vi "Dual_image_snap.vi"() -> ()   [LabVIEW 2013]
uses:
  <vilib>/DAQmx/create/channels.llb/DAQmx Create Channel (CO-Pulse Generation-Frequency).vi
  <vilib>/DAQmx/configure/timing.llb/DAQmx Timing (Implicit).vi
  <vilib>/vision/driver/NI_Vision_Acquisition_Software.lvlib
  <resource>/objmgr/imaqdx.rc
  <resource>/objmgr/daqmx.rc
panel:
  out "Snap Counter":u32
  in  "Snap":bool
  in  "Gain 2":dbl(slide)=575.0 min=350.0 max=1000.0 step=1.0 scale=350.0..1000.0
  in  "VR2":dbl(slide)=65.0 min=0.0 max=255.0 step=1.0 scale=0.0..255.0
  in  "VR1":dbl(slide)=60.0 min=0.0 max=255.0 step=1.0 scale=0.0..255.0
  in  "UB2":dbl(slide)=160.0 min=0.0 max=255.0 step=1.0 scale=0.0..255.0
  in  "UB1":dbl(slide)=165.0 min=0.0 max=255.0 step=1.0 scale=0.0..255.0
  in  "Shutter":dbl(slide)=4095.0 min=0.0 max=4095.0 step=1.0 scale=4.095..4095.0 scale format="%#.0f"
  in  "Brightness":dbl(slide)=100.0 min=0.0 max=255.0 step=1.0 scale=0.0..255.0
  in  "Gain":dbl(slide)=600.0 min=350.0 max=1000.0 step=1.0 scale=350.0..1000.0
  in  "Test Description":string="test"
  in  "Storage Directory":path=path "C:/Users/Regen/Desktop/Users/Ryan Gergely/3D_DIC"
  out "Image 2":T1(plugin-control)
  out "Buffer Number 2":u32
  out "Frame Rate 2":dbl
  in  "Camera Name 2":refnum<k21>="cam2" caption="IMAQdx Session"
  in  "Pule Frequency":dbl=2.0 format="%.1f"
  out "Actual Duty Cycle":dbl
  out "Actual Pulse Frequency":dbl
  in  "Stop":bool
  in  "Start Trigger Mode":bool
  out "Frame Rate 1":dbl
  out "Buffer Number 1":u32
  in  "Camera Name 1":refnum<k21>="cam1" caption="IMAQdx Session"
  out "Image 1":T1(plugin-control)
  # "1) Set Test Description and Storage Directory"
  # "2) Select Cameras"
  # "3) Start VI"
  # "4) Set Frequency and Exposure and White Balance\n(Before Start Trigger)"
  # "5)"
  # "6) Stop When Done"
  # "Exposure Settings - Both Cameras"
  # "White Balance - Camera1"
  # "White Balance - Camera2"
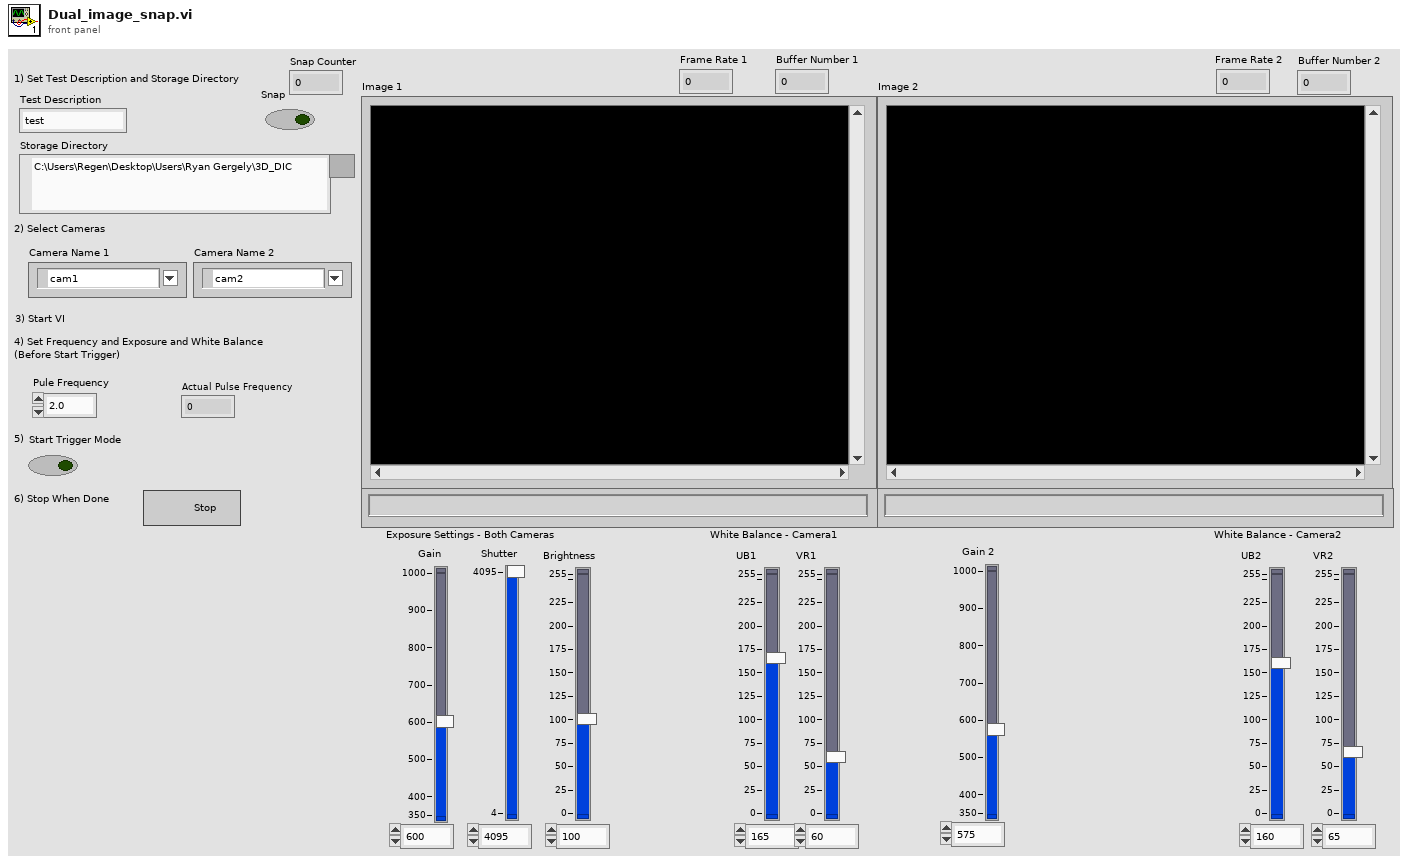
[diagram p1: front panel]
types:
  T1 = typedef "IMAQ Image.ctl" = refnum<image>
  T2 = typedef "IMAQdx.ctl" = refnum<k21>
  T3 = enum16{"open", "replace", "create", "open or create", "replace or create", "replace or create with confirmation"}
  T4 = cluster{"Trigger Mode":u32, "Trigger Activation":u32, "Timeout (ms)":u32}
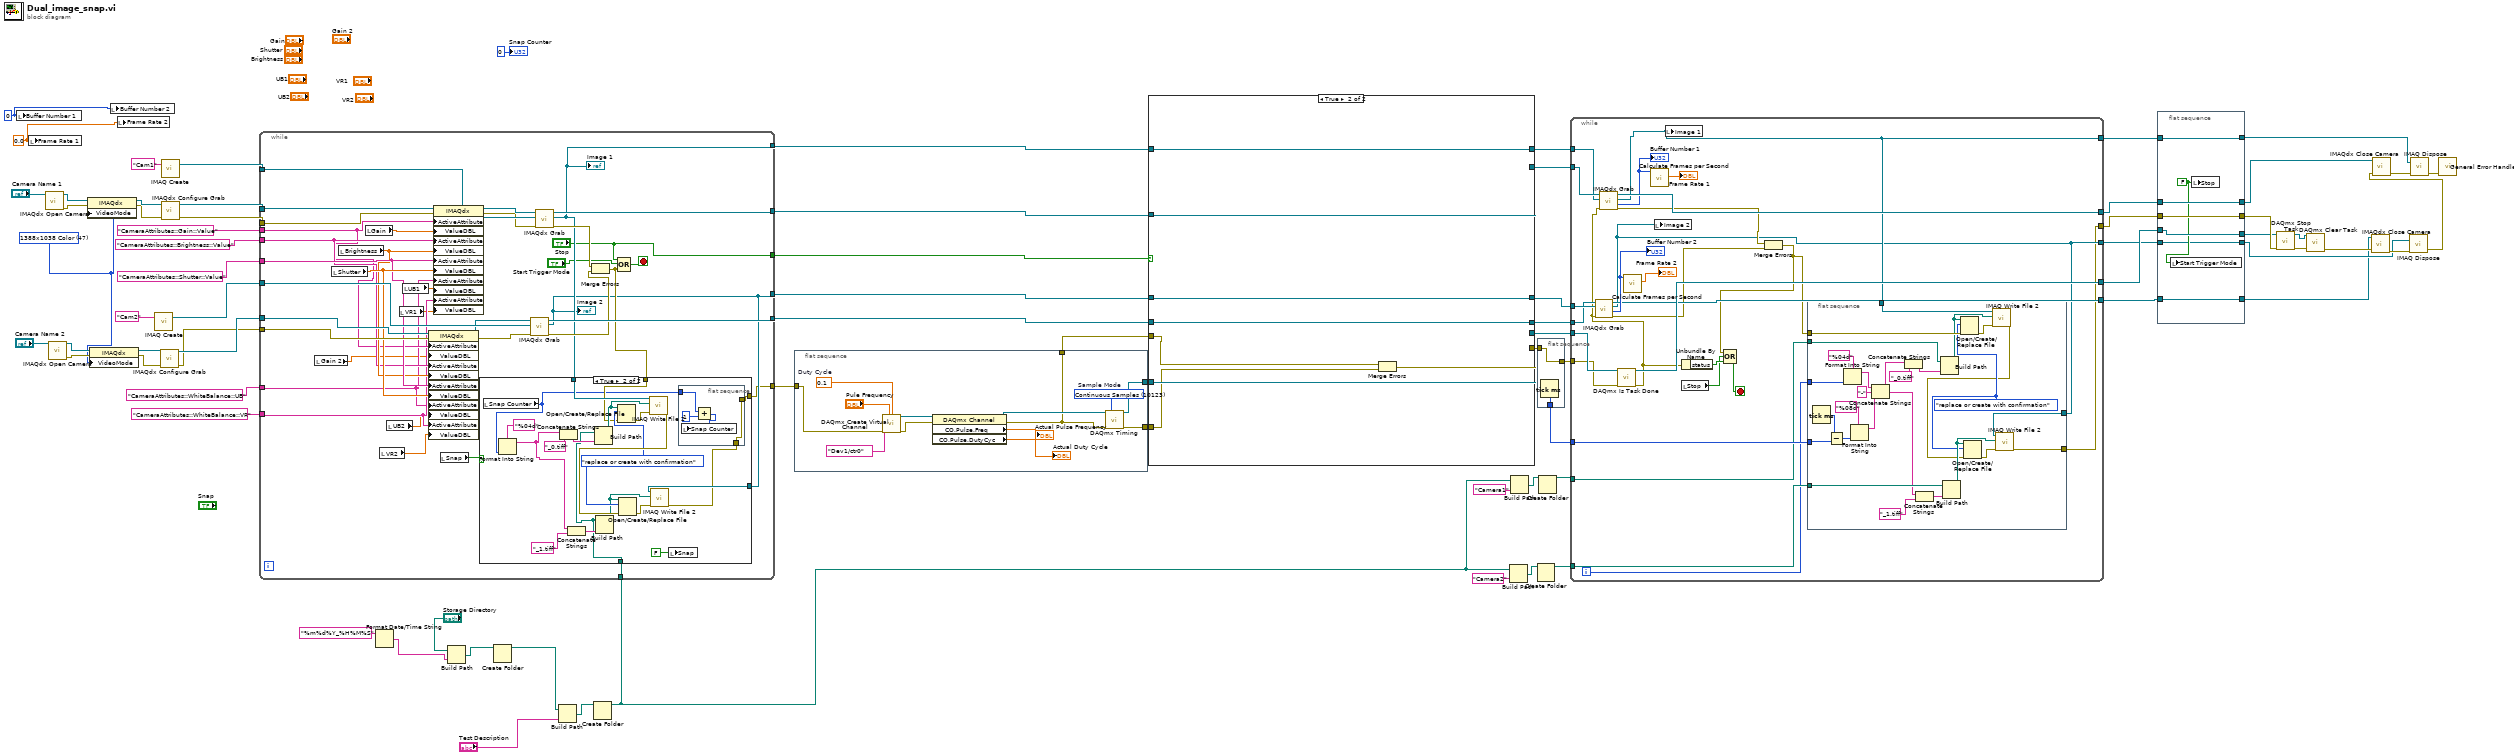
[diagram p0: block diagram]
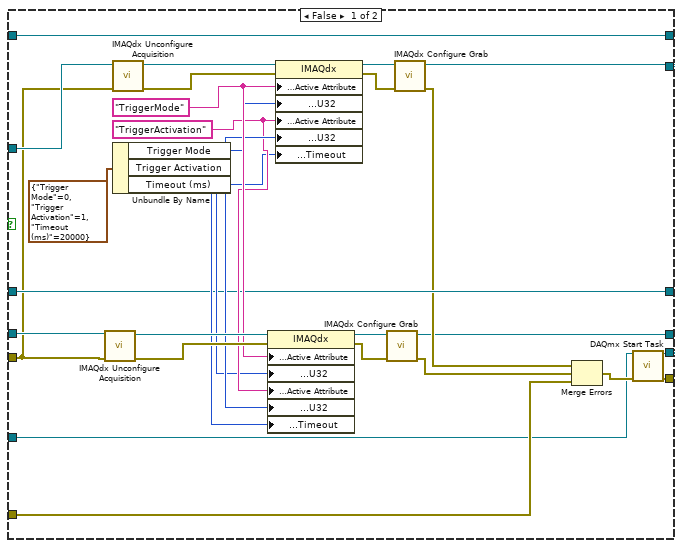
[diagram p2: hidden frame]
diagram:
  w15 = u32 47 items=["320x240 Color"=4, "640x480 Mono8"=9, "640x480 Mono16"=19, "640x480 Color"=14, "800x600 Mono8"=21, "800x600 Mono16"=27, "800x600 Color"=24, "1024x768 Mono8"=30, "1024x768 Mono16"=36, "1024x768 Color"=33, "1280x960 Mono8"=40, "1280x960 Mono16"=46, "1280x960 Color"=43, "1388x1038 Color"=47, "1388x1038 Mono"=48] ("Video Mode")
  w16 = 0.0 ("Frame Rate 1")
  w17 = u32 0 ("Buffer Number 1")
  n1 = local write "Buffer Number 1"(w17) -> ()
  n2 = local write "Frame Rate 1"(w16) -> ()
  n3 = call <vilib>:"IMAQdx Open Camera.vi"("Session In"="Camera Name 1") -> ("error out"=w23:errorcluster, "Session Out"=w25:T2)  [unwired: 2 in, 7 out]
  n4 = call <vilib>:"IMAQdx Open Camera.vi"("Session In"="Camera Name 2") -> ("error out"=w18:errorcluster, "Session Out"=w19:T2)  [unwired: 2 in, 7 out]
  n5 = property class="IMAQdx"(reference=w25, error in=w23, "VideoMode"=w15) -> (reference out=w24:T2, error out=w22:errorcluster)
  n6 = property class="IMAQdx"(reference=w19, error in=w18, "VideoMode"=w15) -> (reference out=w21:T2, error out=w20:errorcluster)
  n7 = local write "Buffer Number 2"(w17) -> ()
  n8 = local write "Frame Rate 2"(w16) -> ()
  n9 = call "IMAQ Create"("Image Name"="Cam2") -> ("New Image"=w13:T1)  [unwired: 3 in, 2 out]
  n10 = call <vilib>:"IMAQdx Configure Grab.vi"("error in"=w20, "Session In"=w21) -> ("error out"=w52:errorcluster, "Session Out"=w53:T2)  [unwired: 8 out]
  n11 = call "IMAQ Create"("Image Name"="Cam1") -> ("New Image"=w63:T1)  [unwired: 3 in, 2 out]
  n12 = call <vilib>:"IMAQdx Configure Grab.vi"("error in"=w22, "Session In"=w24) -> ("error out"=w61:errorcluster, "Session Out"=w62:T2)  [unwired: 8 out]
  n13 = Format Date/Time String(time format string (%c)="%m%d%Y_%H%M%S") -> (date/time string=w35:string)  [unwired: 2 in]
  n14 = Build Path(base path="Storage Directory", name or relative path=w35) -> (appended path=w37:path)
  n15 = Create Folder(path (use dialog)=w37) -> (created path=w4:path)  [unwired: 2 in, 2 out]
  n16 = Build Path(base path=w4, name or relative path="Test Description") -> (appended path=w32:path)
  n17 = Create Folder(path (use dialog)=w32) -> (created path=w1:path)  [unwired: 2 in, 2 out]
  n18 = while {
    tunnel: [w113] -> w74
    tunnel: w61 -> [w107]
    tunnel: w62 -> [w109]
    tunnel: w63 -> [w111]
    tunnel: [w84] -> w58
    tunnel: ["Stop"] -> w59
    tunnel: w53 -> [w105]
    tunnel: w52 -> [w104]
    tunnel: [w112] -> w51
    tunnel: [w82] -> w50
    tunnel: w13 -> [w110]
    tunnel: "CameraAttributes::Shutter::Value" ("ActiveAttribute") -> [w100]
    tunnel: "CameraAttributes::Brightness::Value" ("ActiveAttribute") -> [w98]
    tunnel: "CameraAttributes::Gain::Value" ("ActiveAttribute") -> [w96]
    tunnel: "CameraAttributes::WhiteBalance::UB" ("ActiveAttribute") -> [w93]
    tunnel: "CameraAttributes::WhiteBalance::VR" ("ActiveAttribute") -> [w94]
    tunnel: [w79] -> w3
    tunnel: w1 -> [w78]
    stop <- w88 stop-if-true
    n19 = local read "Gain 2"() -> (w89:dbl)
    n20 = local read "Shutter"() -> (w101:dbl)
    n21 = local read "Brightness"() -> (w99:dbl)
    n22 = local read "Gain"() -> (w97:dbl)
    n23 = local read "VR2"() -> (w90:dbl)
    n24 = local read "UB2"() -> (w92:dbl)
    n25 = local read "VR1"() -> (w91:dbl)
    n26 = local read "UB1"() -> (w95:dbl)
    n27 = property class="IMAQdx"(reference=w105, error in=w104, "ActiveAttribute"=w96, "ValueDBL"=w89, "ActiveAttribute"=w98, "ValueDBL"=w99, "ActiveAttribute"=w100, "ValueDBL"=w101, "ActiveAttribute"=w93, "ValueDBL"=w92, "ActiveAttribute"=w94, "ValueDBL"=w90) -> (reference out=w102:T2, error out=w103:errorcluster)
    n28 = property class="IMAQdx"(reference=w109, error in=w107, "ActiveAttribute"=w96, "ValueDBL"=w97, "ActiveAttribute"=w98, "ValueDBL"=w99, "ActiveAttribute"=w100, "ValueDBL"=w101, "ActiveAttribute"=w93, "ValueDBL"=w95, "ActiveAttribute"=w94, "ValueDBL"=w91) -> (reference out=w108:T2, error out=w106:errorcluster)
    n29 = local read "Snap"() -> (w83:bool)
    n30 = call <vilib>:"IMAQdx Grab.vi"("error in"=w103, "Image In"=w110, "Session In"=w102) -> ("error out"=w87:errorcluster, "Image Out"=w82:T1, "Session Out"=w112:T2)  [unwired: 1 in, 5 out]
    "Image 2" <- w82
    n31 = call <vilib>:"IMAQdx Grab.vi"("error in"=w106, "Image In"=w111, "Session In"=w108) -> ("error out"=w85:errorcluster, "Image Out"=w84:T1, "Session Out"=w113:T2)  [unwired: 1 in, 5 out]
    "Image 1" <- w84
    n32 = Merge Errors(w85, w87) -> (w86:errorcluster)
    n33 = case shown="True" w83 {
      tunnel: w86 -> [w114 w122]
      tunnel: [w114 w117] -> w79
      tunnel: w84 -> [_ w123]
      tunnel: w82 -> [_ w121]
      tunnel: w78 -> [_ w115]
      frame False {
      }
      frame True {
        w126 = T3."replace or create with confirmation" ("operation (0:open)")
        n34 = local read "Snap Counter"() -> (w119:u32)
        n35 = Format Into String(format string="%04d", w119) -> (resulting string=w116:string)  [unwired: 2 in, 1 out]
        n36 = Concatenate Strings(w116, "_0.tiff") -> (w131:string)
        n37 = Concatenate Strings(w116, "_1.tiff") -> (w130:string)
        n38 = Build Path(base path=w115, name or relative path=w131) -> (appended path=w124:path)
        n39 = Build Path(base path=w115, name or relative path=w130) -> (appended path=w125:path)
        n40 = Open/Create/Replace File(file path (use dialog)=w124, error in=w122, operation (0:open)=w126) -> (error out=w127:errorcluster)  [unwired: 3 in, 2 out]
        n41 = call-poly "IMAQ Write File 2"("error in (no error)"=w127, "File Path"=w124, "Image"=w123) -> ("error out"=w129:errorcluster)  [unwired: 7 in, 1 out]
        n42 = Open/Create/Replace File(file path (use dialog)=w125, error in=w129, operation (0:open)=w126) -> (error out=w128:errorcluster)  [unwired: 3 in, 2 out]
        n43 = call-poly "IMAQ Write File 2"("error in (no error)"=w128, "File Path"=w125, "Image"=w121) -> ("error out"=w118:errorcluster)  [unwired: 7 in, 1 out]
        n44 = local write "Snap"(FALSE ("Ready?")) -> ()
        n45 = flat-sequence {
          tunnel: w119 -> [w138]
          tunnel: w118 -> [w135]
          tunnel: [w135] -> w117
          frame #0 {
            n46 = Add(x=w138, y=u32 1) -> (x+y=w136:u32)
            n47 = local write "Snap Counter"(w136) -> ()
          }
        }
      }
    }
    n48 = Compound Arithmetic op=OR("Stop", "Start Trigger Mode", w86) -> (w88:bool)
  }
  n49 = flat-sequence {
    tunnel: [w142] -> w56
    tunnel: [w141] -> w49
    tunnel: w3 -> [w140]
    tunnel: [w139] -> w14
    frame #0 {
      w149 = 0.1  # Duty Cycle
      w143 = 10123 items=["Finite Samples"=10178, "Continuous Samples"=10123, "Hardware Timed Single Point"=12522]  # Sample Mode
      n50 = call-poly <vilib>:"DAQmx Create Virtual Channel.vi"("frequency"="Pule Frequency", "duty cycle"=w149, "counter"=tag "Dev1/ctr0" ("Counter"), "error in"=w140) -> ("task out"=w145:refnum<k21>, "error out"=w146:errorcluster)  [unwired: 10 in]
      n51 = property class="DAQmx Channel"(reference=w145, error in=w146) -> (reference out=w147:refnum<k21>, error out=w139:errorcluster, "CO.Pulse.Freq"=→"Actual Pulse Frequency":dbl, "CO.Pulse.DutyCyc"=→"Actual Duty Cycle":dbl)
      n52 = call-poly <vilib>:"DAQmx Timing.vi"("task/channels in"=w147, "sample mode"=w143, "error in"=w139) -> ("task out"=w142:refnum<k21>, "error out"=w141:errorcluster)  [unwired: 11 in]
    }
  }
  n53 = case shown="True" w59 {
    tunnel: w74 -> [w179 w187]
    tunnel: [w178 w187] -> w73
    tunnel: [w160 w184] -> w7
    tunnel: [w161 w185] -> w71
    tunnel: w58 -> [w172 w186]
    tunnel: [w172 w186] -> w57
    tunnel: w56 -> [w153 w185]
    tunnel: w14 -> [w152 w183]
    tunnel: w51 -> [w163 w180]
    tunnel: w50 -> [w162 w181]
    tunnel: [w162 w181] -> w48
    tunnel: w49 -> [w156 w182]
    tunnel: [w154 w180] -> w47
    frame False {
      w166 = "TriggerActivation" ("ActiveAttribute")
      w168 = "TriggerMode" ("ActiveAttribute")
      n54 = call <vilib>:"IMAQdx Unconfigure Acquisition.vi"("error in"=w152, "Session In"=w163) -> ("error out"=w170:errorcluster, "Session Out"=w169:T2)  [unwired: 8 out]
      n55 = call <vilib>:"IMAQdx Unconfigure Acquisition.vi"("error in"=w152, "Session In"=w179) -> ("error out"=w175:errorcluster, "Session Out"=w174:T2)  [unwired: 8 out]
      n56 = Unbundle By Name(T4 {"Trigger Mode"=0, "Trigger Activation"=1, "Timeout (ms)"=20000} ("Trigger Parameters")) -> ("Trigger Mode"=w164:u32, "Trigger Activation"=w167:u32, "Timeout (ms)"=w165:u32)
      n57 = property class="IMAQdx"(reference=w169, error in=w170, "Camera Attributes:Active Attribute"=w168, "Camera Attributes:Value:U32"=w164, "Camera Attributes:Active Attribute"=w166, "Camera Attributes:Value:U32"=w167, "Acquisition Attributes:Timeout"=w165) -> (reference out=w171:T2, error out=w159:errorcluster)
      n58 = property class="IMAQdx"(reference=w174, error in=w175, "Camera Attributes:Active Attribute"=w168, "Camera Attributes:Value:U32"=w164, "Camera Attributes:Active Attribute"=w166, "Camera Attributes:Value:U32"=w167, "Acquisition Attributes:Timeout"=w165) -> (reference out=w176:T2, error out=w177:errorcluster)
      n59 = call <vilib>:"IMAQdx Configure Grab.vi"("error in"=w159, "Session In"=w171) -> ("error out"=w157:errorcluster, "Session Out"=w154:T2)  [unwired: 8 out]
      n60 = call <vilib>:"IMAQdx Configure Grab.vi"("error in"=w177, "Session In"=w176) -> ("error out"=w155:errorcluster, "Session Out"=w178:T2)  [unwired: 8 out]
      n61 = Merge Errors(w155, w157, w156) -> (w158:errorcluster)
      n62 = call <vilib>:"DAQmx Start Task.vi"("task/channels in"=w153, "error in"=w158) -> ("task out"=w161:refnum<k21>, "error out"=w160:errorcluster)  [unwired: 12 in]
    }
    frame True {
      n63 = Merge Errors(w183, w182) -> (w184:errorcluster)
    }
  }
  n64 = Build Path(base path=w1, name or relative path="Camera2") -> (appended path=w27:path)
  n65 = Build Path(base path=w1, name or relative path="Camera1") -> (appended path=w30:path)
  n66 = flat-sequence {
    tunnel: w7 -> [w189]
    tunnel: [w189] -> w6
    tunnel: [w188] -> w5
    frame #0 {
      n67 = Tick Count (ms)() -> (millisecond timer value=w188:u32)
    }
  }
  n68 = Create Folder(path (use dialog)=w27) -> (created path=w26:path)  [unwired: 2 in, 2 out]
  n69 = Create Folder(path (use dialog)=w30) -> (created path=w29:path)  [unwired: 2 in, 2 out]
  n70 = while {
    tunnel: [w216] -> w67
    tunnel: [w194] -> w68
    tunnel: w73 -> [w213]
    tunnel: w57 -> [w212]
    tunnel: [w209] -> w69
    tunnel: w71 -> [w208]
    tunnel: w48 -> [w205]
    tunnel: w47 -> [w204]
    tunnel: w6 -> [w201]
    tunnel: [w198] -> w39
    tunnel: [w197] -> w43
    tunnel: [w200] -> w41
    tunnel: w29 -> [w191]
    tunnel: w26 -> [w199]
    tunnel: w5 -> [w193]
    i -> [w190]
    stop <- w210 stop-if-true
    n71 = call <vilib>:"DAQmx Is Task Done.vi"("task/channels in"=w208, "error in"=w201) -> ("task out"=w209:refnum<k21>, "error out"=w195:errorcluster)  [unwired: 11 in, 1 out]
    n72 = call <vilib>:"IMAQdx Grab.vi"("error in"=w195, "Image In"=w205, "Session In"=w204) -> ("error out"=w196:errorcluster, "Buffer Number Out"=w203:u32, "Image Out"=w197:T1, "Session Out"=w200:T2)  [unwired: 1 in, 4 out]
    "Buffer Number 2" <- w203
    n73 = call <vilib>:"IMAQdx Grab.vi"("error in"=w195, "Image In"=w212, "Session In"=w213) -> ("error out"=w202:errorcluster, "Buffer Number Out"=w214:u32, "Image Out"=w198:T1, "Session Out"=w216:T2)  [unwired: 1 in, 4 out]
    "Buffer Number 1" <- w214
    n74 = call <vilib>:"Calculate Frames per Second.vi"("Buffer Number"=w203) -> ("Processed Frames/s"=→"Frame Rate 2":dbl)  [unwired: 8 in, 2 out]
    n75 = call <vilib>:"Calculate Frames per Second.vi"("Buffer Number"=w214) -> ("Processed Frames/s"=→"Frame Rate 1":dbl)  [unwired: 8 in, 2 out]
    n76 = local write "Image 2"(w197) -> ()
    n77 = local write "Image 1"(w198) -> ()
    n78 = Unbundle By Name(w195) -> ("status"=w211:bool)
    n79 = local read "Stop"() -> (w207:bool)
    n80 = Merge Errors(w202, w196) -> (w192:errorcluster)
    n81 = Compound Arithmetic op=OR(w192, w207, w211) -> (w210:bool)
    n82 = flat-sequence {
      tunnel: w191 -> [w242]
      tunnel: w199 -> [w241]
      tunnel: w198 -> [w240]
      tunnel: w197 -> [w239]
      tunnel: w192 -> [w238]
      tunnel: [w237] -> w194
      tunnel: w193 -> [w230]
      tunnel: w190 -> [w222]
      frame #0 {
        w234 = T3."replace or create with confirmation" ("operation (0:open)")
        n83 = Tick Count (ms)() -> (millisecond timer value=w229:u32)
        n84 = Subtract(x=w229, y=w230) -> (x-y=w225:u32)
        n85 = Format Into String(format string="%04d", w222) -> (resulting string=w220:string)  [unwired: 2 in, 1 out]
        n86 = Format Into String(format string="%08d", w225) -> (resulting string=w224:string)  [unwired: 2 in, 1 out]
        n87 = Concatenate Strings(w220, "-" ("string"), w224) -> (w217:string)
        n88 = Concatenate Strings(w217, "_0.tiff") -> (w227:string)
        n89 = Concatenate Strings(w217, "_1.tiff") -> (w228:string)
        n90 = Build Path(base path=w242, name or relative path=w227) -> (appended path=w236:path)
        n91 = Build Path(base path=w241, name or relative path=w228) -> (appended path=w235:path)
        n92 = Open/Create/Replace File(file path (use dialog)=w236, error in=w238, operation (0:open)=w234) -> (error out=w233:errorcluster)  [unwired: 3 in, 2 out]
        n93 = call-poly "IMAQ Write File 2"("error in (no error)"=w233, "File Path"=w236, "Image"=w240) -> ("error out"=w231:errorcluster)  [unwired: 7 in, 1 out]
        n94 = Open/Create/Replace File(file path (use dialog)=w235, error in=w231, operation (0:open)=w234) -> (error out=w232:errorcluster)  [unwired: 3 in, 2 out]
        n95 = call-poly "IMAQ Write File 2"("error in (no error)"=w232, "File Path"=w235, "Image"=w239) -> ("error out"=w237:errorcluster)  [unwired: 7 in, 1 out]
      }
    }
  }
  n96 = flat-sequence {
    tunnel: w69 -> [w247]
    tunnel: w68 -> [w248]
    tunnel: w67 -> [w249]
    tunnel: [w249] -> w66
    tunnel: [w248] -> w65
    tunnel: [w247] -> w64
    tunnel: [w245] -> w42
    tunnel: w43 -> [w245]
    tunnel: w41 -> [w244]
    tunnel: [w244] -> w40
    tunnel: w39 -> [w243]
    tunnel: [w243] -> w38
    frame #0 {
      w246 = FALSE ("Stop")
      n97 = local write "Start Trigger Mode"(w246) -> ()
      n98 = local write "Stop"(w246) -> ()
    }
  }
  n99 = call <vilib>:"DAQmx Stop Task.vi"("task/channels in"=w64, "error in"=w65) -> ("task out"=w70:refnum<k21>, "error out"=w72:errorcluster)  [unwired: 12 in]
  n100 = call <vilib>:"DAQmx Clear Task.vi"("task in"=w70, "error in"=w72) -> ("error out"=w44:errorcluster)  [unwired: 13 in]
  n101 = call <vilib>:"IMAQdx Close Camera.vi"("error in"=w44, "Session In"=w40) -> ("error out"=w46:errorcluster)  [unwired: 9 out]
  n102 = call "IMAQ Dispose"("Image"=w42, "error in (no error)"=w46) -> ("error out"=w45:errorcluster)  [unwired: 4 in]
  n103 = call <vilib>:"IMAQdx Close Camera.vi"("error in"=w45, "Session In"=w66) -> ("error out"=w77:errorcluster)  [unwired: 9 out]
  n104 = call "IMAQ Dispose"("Image"=w38, "error in (no error)"=w77) -> ("error out"=w76:errorcluster)  [unwired: 4 in]
  n105 = call <vilib>:"General Error Handler.vi"("error in (no error)"=w76) -> ()  [unwired: 1 in, 14 out]
  "Snap Counter" <- u32 0 ("Snap Counter")
